vi "send_vehicle_command_wait.vi"(2 "Brake":bool, 3 "Drive mode":bool, 4 "error in":errorcluster, 5 "Right amount":dbl, 6 "Forward amount":dbl) -> (0 "error out":errorcluster)   [LabVIEW 2019, in "Lib_Simx.lvlib"]
doc: "Sends a command to the Simulator to control the movement of ego vehicle.\n Parameters:\n -- forward_amount: a value between -1.0 and 1.0 that determines the amount of throttle to apply\n -- right_amount: a value between -1.0 and 1.0 that determines the steering position (-1 is left, +1 is right)"
uses:
  Lib_Simx.lvlib
  tools/simx_common.vi
panel:
  out "success":bool
  out "TCP Network Connection out":refnum<k5>
  out "Vehicle command response":string
  # "Overview: Sends a command to the monoDrive Simulator to control the movement of ego vehicle.\n Parameters:\n  -- forward_amount: a value between -1.0 and 1.0 that determines the amount of throttle to apply\n  -- right_amount: a value between -1.0 and 1.0 that determines the steering position (-1 is left, +1 is right)\nInstructions:\nThe command used to control the throttle (forward_amount) and steering (right_amount) is used to move the ego vehicle inside the simulation. The response from the simulator will appear in the vehicle command response field below."
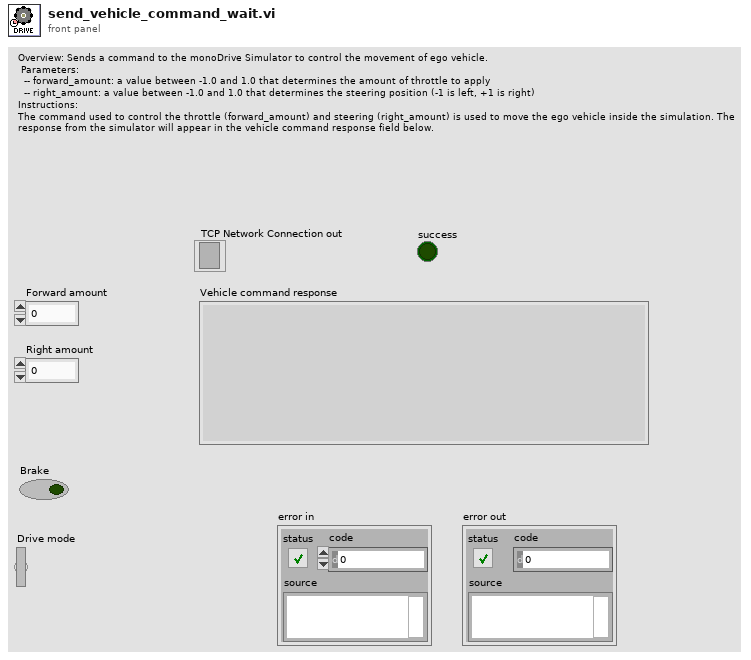
[diagram p1: front panel]
types:
  T1 = typedef "Lib_Simx.lvlib/simx_connection.ctl" = cluster{"Config":T2, "Connections":T5, "Map":cluster{"lanes":cluster{"x":dbl[], "y":dbl[], "z":dbl[]}, "StartPosition":cluster{"start_points":T6, "StartRotation":dbl[], "StartLocation":dbl[]}, "Draw Map Size":T7, "DrawArea":cluster{"min_Y":dbl, "min_X":dbl, "Scale X":dbl, "Scale Y":dbl}, "Map":picture, "Map Geojson":string}}
  T2 = typedef "Lib_Simx.lvlib/config.ctl" = cluster{"Trajectory":T3, "Weather":T4}
  T3 = typedef "Lib_Simx.lvlib/trajectory.ctl" = cluster{"Number of frames":i32, "Frame number":i32, "Trajectory":string}
  T4 = typedef "Lib_Simx.lvlib/weather.ctl" = cluster{"id":string}
  T5 = typedef "Lib_Simx.lvlib/connections.ctl" = cluster{"Simulator Connection":refnum<k5>, "server_ip":string, "Port":i32, "Sensor connections":refnum<k5>[]}
  T6 = typedef "Lib_Simx.lvlib/start_points.ctl" = cluster{"locations":dbl[][], "rotations":dbl[][], "type":string[]}
  T7 = typedef "LVBoundsTypeDef.ctl" = cluster{"Width":u32, "Height":u32}
  T8 = cluster{"forward_amount":dbl, "right_amount":dbl, "brake_amount":i16, "drive_mode":i16}
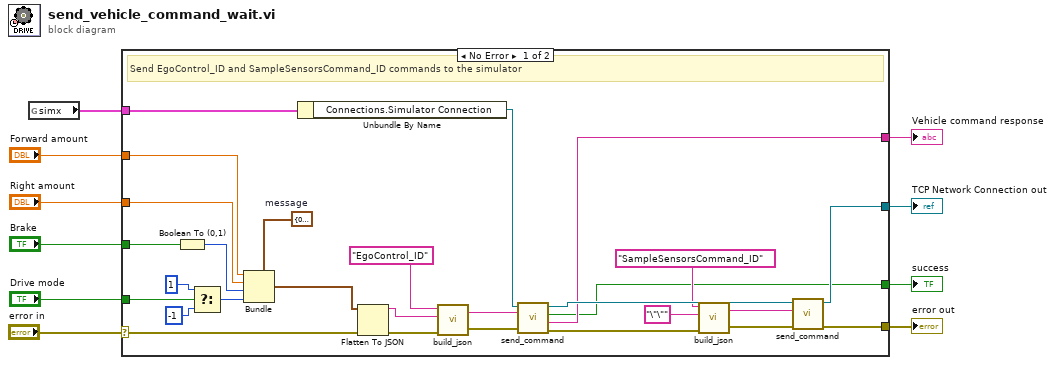
[diagram p0: block diagram]
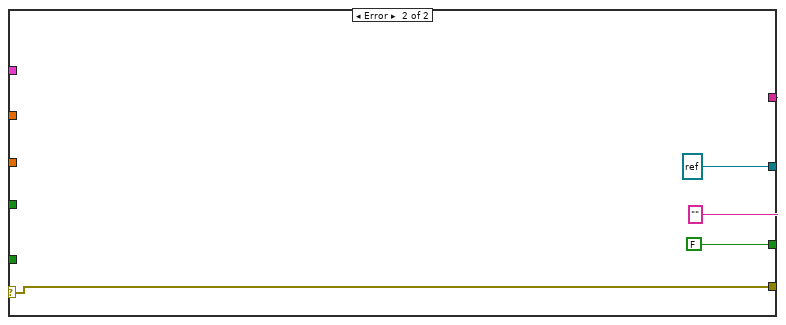
[diagram p2: hidden frame]
diagram:
  n1 = global read "simx_common.vi" "simx"() -> (w1:T1)
  n2 = case shown="No Error" "error in" {
    selector: "error in" -> [w12 w42]
    tunnel: [w24 w42] -> w10
    tunnel: "Right amount" -> [w38 _]
    tunnel: "Forward amount" -> [w37 _]
    tunnel: [w20 "" ("response")] -> w7
    tunnel: [w23 refnum<k5> refnum ("TCP Network Connection Out")] -> w6
    tunnel: [w11 FALSE ("success")] -> w5
    tunnel: "Brake" -> [w35 _]
    tunnel: "Drive mode" -> [w34 _]
    tunnel: w1 -> [w30 _]
    frame No Error {
      w13 = T8 {"forward_amount"=0.0, "right_amount"=0.0, "brake_amount"=0, "drive_mode"=0}  # message
      # "Send EgoControl_ID and SampleSensorsCommand_ID commands to the simulator"
      n3 = Boolean To (0,1)(Boolean=w35) -> (0, 1=w36:i16)
      n4 = Select(t=1, s=w34, f=-1) -> (s? t:f=w31:i32)
      n5 = Bundle(cluster=w13, "forward_amount"=w37, "right_amount"=w38, "brake_amount"=w36, "drive_mode"=w31) -> (w17:T8)
      n6 = Unbundle By Name(w30) -> ("Connections.Simulator Connection"=w28:refnum<k5>)
      n7 = Flatten To JSON(anything=w17, error in (no error)=w12) -> (JSON string=w15:string, 11:w16:errorcluster)  [unwired: 1 in]
      n8 = call "build_json.vi"("error in"=w16, "Message"=w15, "Command_ID"="EgoControl_ID") -> ("error out"=w29:errorcluster, "JSON Out"=w27:string)  [unwired: 1 in]
      n9 = call "send_command.vi"("error in"=w29, "JSON Command"=w27, "TCP Network Connection in"=w28) -> ("error out"=w26:errorcluster, "Response"=w20:string, "Success"=w11:bool, "TCP Network Connection Out"=w21:refnum<k5>)  [unwired: 1 in]
      n10 = call "build_json.vi"("error in"=w26, "Message"="\"\"" ("message"), "Command_ID"="SampleSensorsCommand_ID" ("type")) -> ("error out"=w25:errorcluster, "JSON Out"=w22:string)  [unwired: 1 in]
      n11 = call "send_command.vi"("error in"=w25, "JSON Command"=w22, "TCP Network Connection in"=w21) -> ("error out"=w24:errorcluster, "TCP Network Connection Out"=w23:refnum<k5>)  [unwired: 1 in, 2 out]
    }
    frame Error {
    }
  }
  "Vehicle command response" <- w7
  "TCP Network Connection out" <- w6
  "error out" <- w10
  "success" <- w5
